vi "Line+Scan_Y.vi"() -> ()   [LabVIEW 2014]
doc: "This is the main user interface of the Raman spectroscopy system."
uses:
  <userlib>/atmcd64d.llb/AcquisitionMode_mode typedef.ctl
  <userlib>/atmcd64d.llb/ReadMode_mode typedef.ctl
  <userlib>/atmcd64d.llb/Shutter_mode typedef.ctl
  <userlib>/atmcd64d.llb/Shutter_type typedef.ctl
  <userlib>/atmcd64d.llb/TriggerMode_mode typedef.ctl
  TypeDef/GalvoInput.ctl
  <userlib>/atmcd64d.llb/Error Code Enum typedef.ctl
  TypeDef/States.ctl
panel:
  in  "Tab Control":enum32{"Main", "Andor", "Galvo"}(tab)
  in  "Galvo Center":bool
  out "Galvo":bool
  in  "Quit":bool
  out "Initialization finished":bool
  in  "Galvo Stop":bool
  in  "Galvo Scan":bool
  out "Andor":bool
  out "CurrentFrame":i32
  in  "Scan parameters":T1={"area/um"=10.2262, "range_x/v"=0.17651, "range_y/v"=0.2155, "interval/um"=0.15978, "x_center/v"=3.35, "y_center/v"=5.55, "theta_1/de"=0.0, "theta_2/de"=60.0, "theta_3/de"=120.0}
  in  "Set":bool
  in  "AndorSnap":bool
  out "SaveStatus":bool
  in  "FilePath":string="C:\\Users\\light\\Desktop\\SI+Raman\\data\\TEMP"
  in  "Exit":bool
  out "ShutDown":cluster{"CoolOff":bool, "ShutDown":bool}
  in  "Mode":T7={"AcqMode"=enum."Single Scan", "ReadMode"=enum."Image", "ShutterMode"=enum."Auto", "GateMode"=enum."TTL High", "TriggerMode"=enum."Internal"}
  in  "AcqSet":T8={"openingtime"=0, "closingtime/ms"=10, "ExposureTime/s"=10.0, "AccumCycTime"=0.0, "AccumCycNum"=1, "KineticNum"=1, "KineticTime"=0.0} {"KineticTime" format="%.5f"; "AccumCycNum" format="%.5f"; "AccumCycTime" format="%.5f"; "ExposureTime/s" format="%.5f"; "closingtime/ms" format="%.2f"; "openingtime" format="%.2f"}
  out "Timing":T9 {"kinetic" format="%.7f"; "accumulate" format="%.7f"; "exposure" format="%.7f"}
  out "SetOut":T10
  in  "MultiTrack":cluster{"StartRow":i32, "EndRow":i32}={"StartRow"=131, "EndRow"=143}
  out "SetStatus":bool
  out "CurrentTemp":i32
  out "DevInit":bool
  out "DevSize":cluster{"xpixels":i32, "ypixels":i32}
  out "HardWVersion":T11
  out "SoftWVersion":T12
  out "Speeds":T13
  in  "TargetTemp":i32=-60
  out "CoolerON":T14
  out "GetStatus":T15
  in  "YOffset":dbl=5.75 caption="Offset"
  in  "XOffset":dbl=3.1 caption="Offset"
  out "Sample Rate":dbl=1000.0 format="%0.2f"
  out "Waveform Graph":waveform(dbl)[](graph)=[{"t0"=timestamp(0 s since 1904-01-01), "dt"=0.001, "Y"=[]}]
  in  "ZOffset":dbl=1.6 caption="Offset"
  in  "Galvo":T16={"Sample Rate"=1000000.0, "Sample Clock Source"="OnboardClock", "Max Voltage"=10.0, "Min Voltage"=-10.0, "Physical Channel(s)"="Dev1/ao0,Dev1/ao1,Dev1/ao3"}
  in  "Reset":bool
  # "Objective: CFI Plan Fluor ELWD 60x (1.27 NA) \nThe depth of field: 1.78 um\nPixel Size: 0.0877um/px"
  # "Kinetics->SignleTrack"
  # "Galvo Control"
  # "10^4->1s"
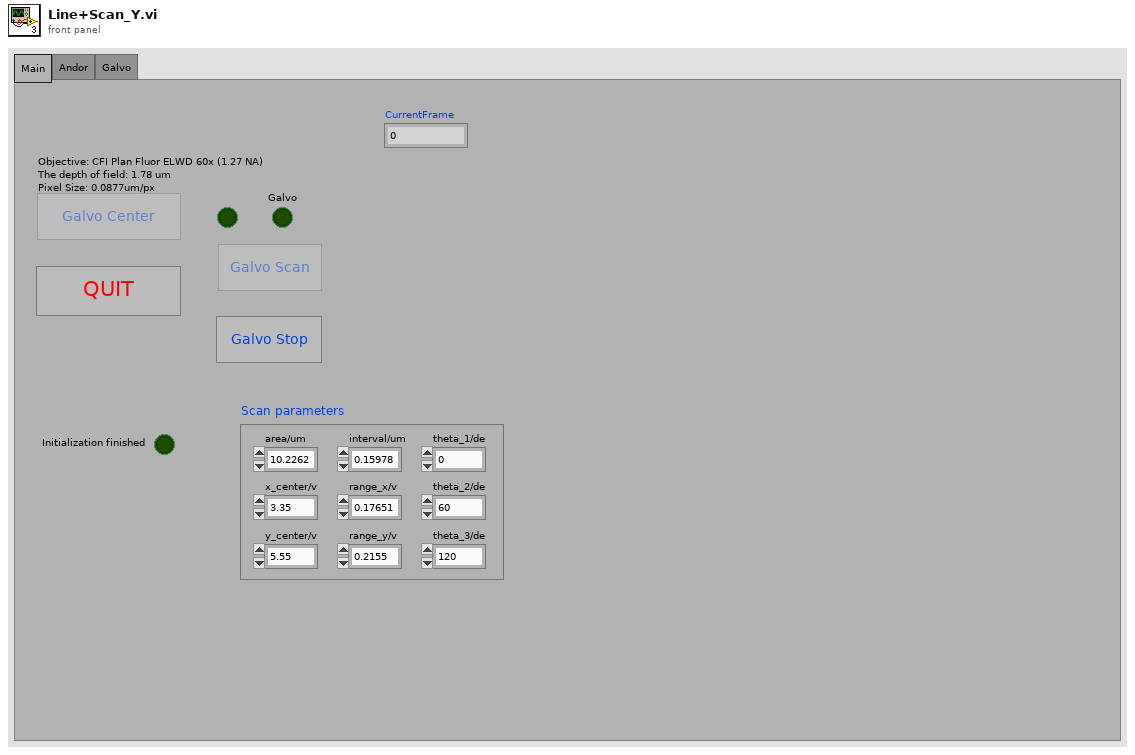
[diagram p1: front panel]
types:
  T1 = cluster{"area/um":dbl, "range_x/v":dbl, "range_y/v":dbl, "interval/um":dbl, "x_center/v":dbl, "y_center/v":dbl, "theta_1/de":dbl, "theta_2/de":dbl, "theta_3/de":dbl}
  T2 = typedef "AcquisitionMode_mode typedef.ctl" = enum16{"Reserved (0)", "Single Scan", "Accumulate", "Kinetics", "Fast Kinetics", "Run Till Abort", "Reserved (6)", "Reserved (7)", "Reserved (8)", "Time Delayed Integration"}
  T3 = typedef "ReadMode_mode typedef.ctl" = enum16{"Full Vertical Binning", "Multi-Track", "Random-Track", "Single-Track", "Image"}
  T4 = typedef "Shutter_mode typedef.ctl" = enum16{"Auto", "Open", "Close", "N/A (3)", "Open FVB Series", "Open Any Series"}
  T5 = typedef "Shutter_type typedef.ctl" = enum16{"TTL Low", "TTL High"}
  T6 = typedef "TriggerMode_mode typedef.ctl" = enum16{"Internal", "External", "N/A (2)", "N/A (3)", "N/A (4)", "N/A (5)", "External Start", "External Exposure (Bulb)", "N/A (8)", "External FVB EM", "Software", "N/A (11)", "External Charge Shifting"}
  T7 = cluster{"AcqMode":T2, "ReadMode":T3, "ShutterMode":T4, "GateMode":T5, "TriggerMode":T6}
  T8 = cluster{"openingtime":i32, "closingtime/ms":i32, "ExposureTime/s":sgl, "AccumCycTime":sgl, "AccumCycNum":i32, "KineticNum":i32, "KineticTime":sgl}
  T9 = cluster{"exposure":sgl, "accumulate":sgl, "kinetic":sgl}
  T10 = cluster{"Height":i32, "Width":i32, "bottom":i32, "gap":i32}
  T11 = cluster{"PCB":u32, "Flex":u32, "dummy1":u32, "dummy2":u32, "dummy3":u32, "dummy4":u32}
  T12 = cluster{"eprom":u32, "cofFile":u32, "vxdRev":u32, "vxdVer":u32, "dllRev":u32, "dllVer":u32}
  T13 = cluster{"NVS":i32, "VS":i32, "NHS":dbl, "HS":i32}
  T14 = cluster{"SetTemp":bool, "CoolerOn":bool, "Stablized":bool}
  T15 = cluster{"GetDetector":bool, "GetHardVer":bool, "GetNVS":bool, "GetVS":bool, "GetSotfVer":bool, "GetNHS":bool, "GetHS":bool}
  T16 = typedef "GalvoInput.ctl" = cluster{"Sample Rate":dbl, "Sample Clock Source":tag, "Max Voltage":dbl, "Min Voltage":dbl, "Physical Channel(s)":tag}
  T17 = typedef "States.ctl" = enum16{"Initialize", "CMOS live", "Shut down"}
  T18 = enum8{"Enabled", "Disabled", "Disabled and Grayed Out"}
  T19 = typedef "Error Code Enum typedef.ctl" = enum32{"N/A (0)", "DRV_ERROR_CODES", "DRV_SUCCESS", "DRV_VXDNOTINSTALLED", "DRV_ERROR_SCAN", "DRV_ERROR_CHECK_SUM", "DRV_ERROR_FILELOAD", "DRV_UNKNOWN_FUNC", "DRV_ERROR_VXD_INIT", "DRV_ERROR_ADDRESS", "DRV_ERROR_PAGELOCK", "DRV_ERROR_PAGEUNLOCK", "DRV_ERROR_BOARDTEST", "DRV_ERROR_ACK", "DRV_ERROR_UP_FIFO", "DRV_ERROR_PATTERN", "N/A (16)", "DRV_ACQUISITION_ERRORS", "DRV_ACQ_BUFFER", "DRV_ACQ_DOWNFIFO_FULL", "DRV_PROC_UNKONWN_INSTRUCTION", "DRV_ILLEGAL_OP_CODE", "DRV_KINETIC_TIME_NOT_MET", "DRV_ACCUM_TIME_NOT_MET", "DRV_NO_NEW_DATA", "N/A (25)", "DRV_SPOOLERROR", "N/A (27)", "N/A (28)", "N/A (29)", "N/A (30)", "N/A (31)", "N/A (32)", "DRV_TEMPERATURE_CODES", "DRV_TEMPERATURE_OFF", "DRV_TEMPERATURE_NOT_STABILIZED", "DRV_TEMPERATURE_STABILIZED", "DRV_TEMPERATURE_NOT_REACHED", "DRV_TEMPERATURE_OUT_RANGE", "DRV_TEMPERATURE_NOT_SUPPORTED", "DRV_TEMPERATURE_DRIFT", "N/A (41)", "N/A (42)", "N/A (43)", "N/A (44)", "N/A (45)", "N/A (46)", "N/A (47)", "N/A (48)", "DRV_GENERAL_ERRORS", "DRV_INVALID_AUX", "DRV_COF_NOTLOADED", "DRV_FPGAPROG", "DRV_FLEXERROR", "DRV_GPIBERROR", "N/A (55)", "N/A (56)", "N/A (57)", "N/A (58)", "N/A (59)", "N/A (60)", "N/A (61)", "N/A (62)", "N/A (63)", "DRV_DATATYPE", "DRV_DRIVER_ERRORS", "DRV_P1INVALID", "DRV_P2INVALID", "DRV_P3INVALID", "DRV_P4INVALID", "DRV_INIERROR", "DRV_COFERROR", "DRV_ACQUIRING", "DRV_IDLE", "DRV_TEMPCYCLE", "DRV_NOT_INITIALIZED", "DRV_P5INVALID", "DRV_P6INVALID", "DRV_INVALID_MODE", "DRV_INVALID_FILTER", "DRV_I2CERRORS", "DRV_I2CDEVNOTFOUND", "DRV_I2CTIMEOUT", "DRV_P7INVALID", "N/A (84)", "N/A (85)", "N/A (86)", "N/A (87)", "N/A (88)", "N/A (89)", "DRV_IOCERROR", "DRV_VRMVERSIONERROR"}
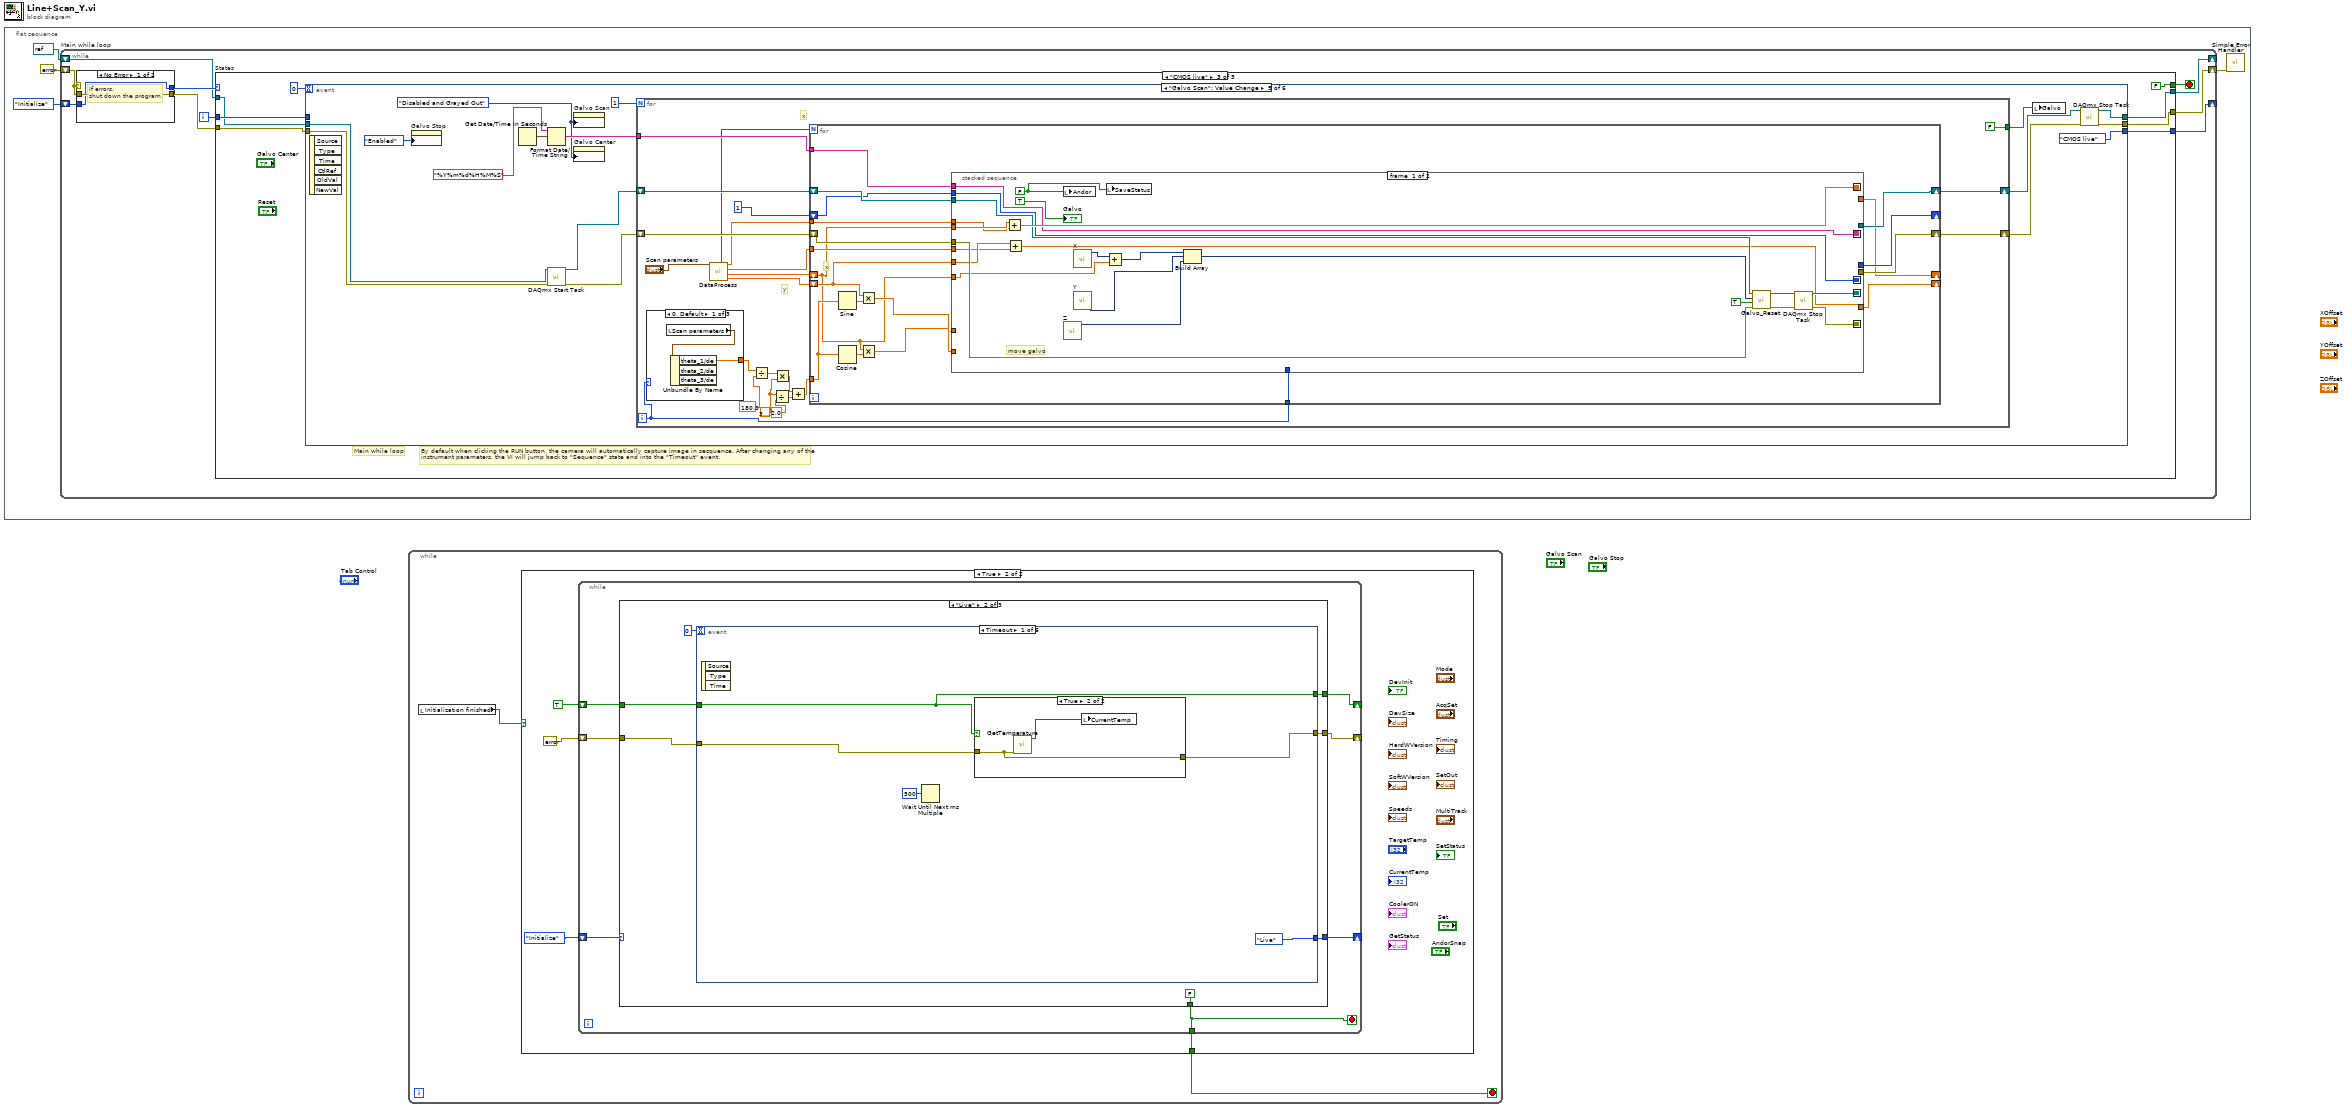
[diagram p0: block diagram]
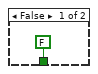
[diagram p2: hidden frame]
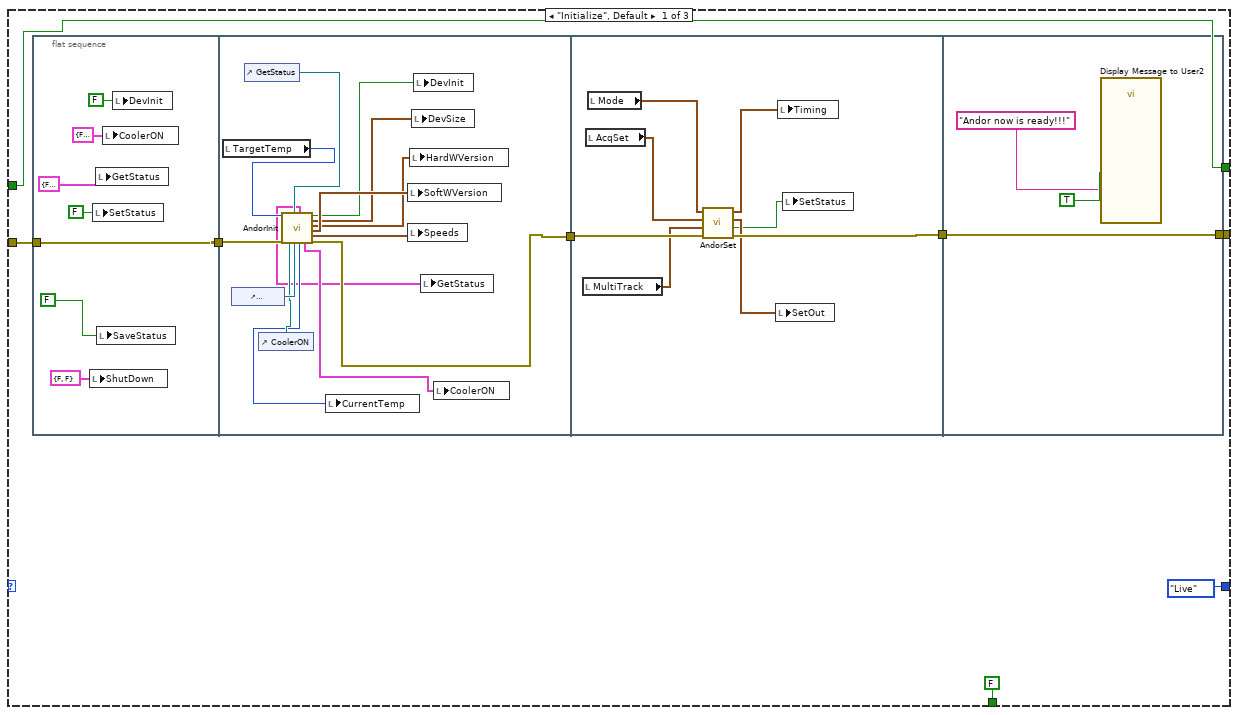
[diagram p3: hidden frame]
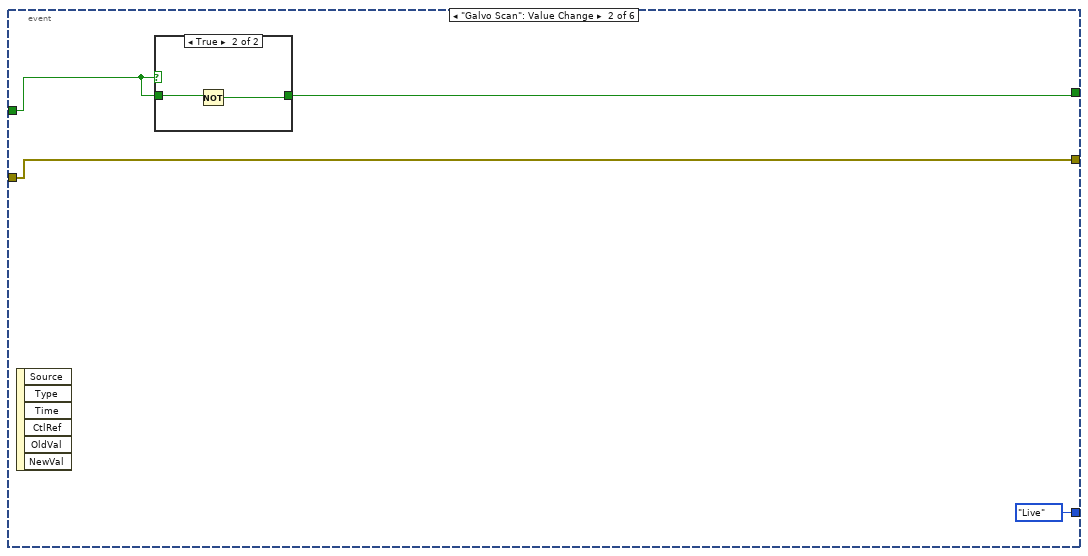
[diagram p5: hidden frame]
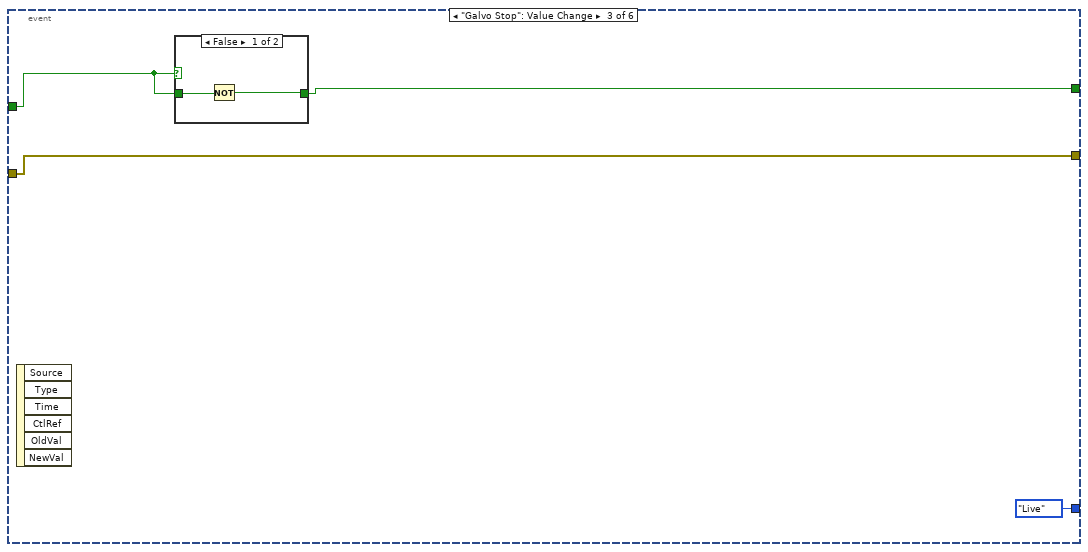
[diagram p7: hidden frame]
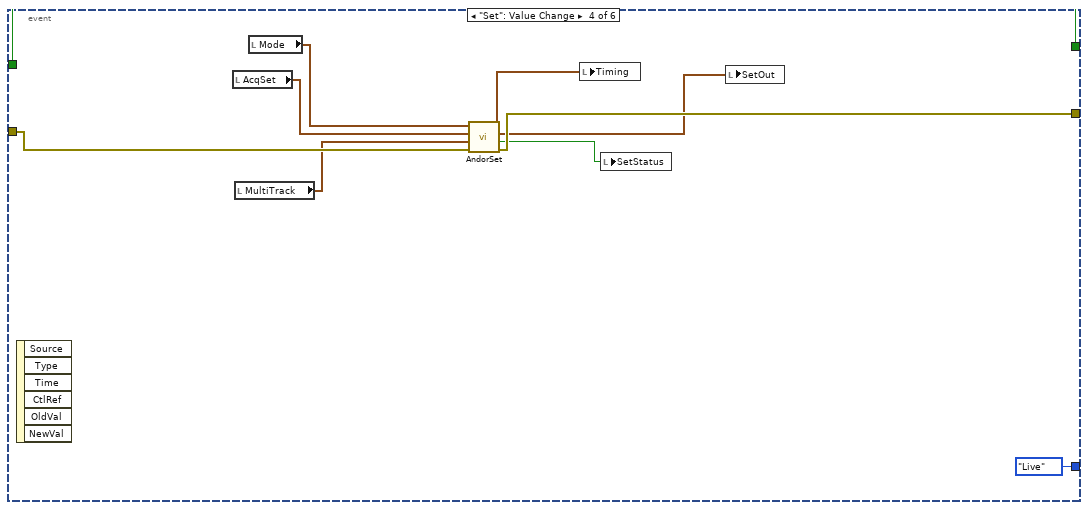
[diagram p9: hidden frame]
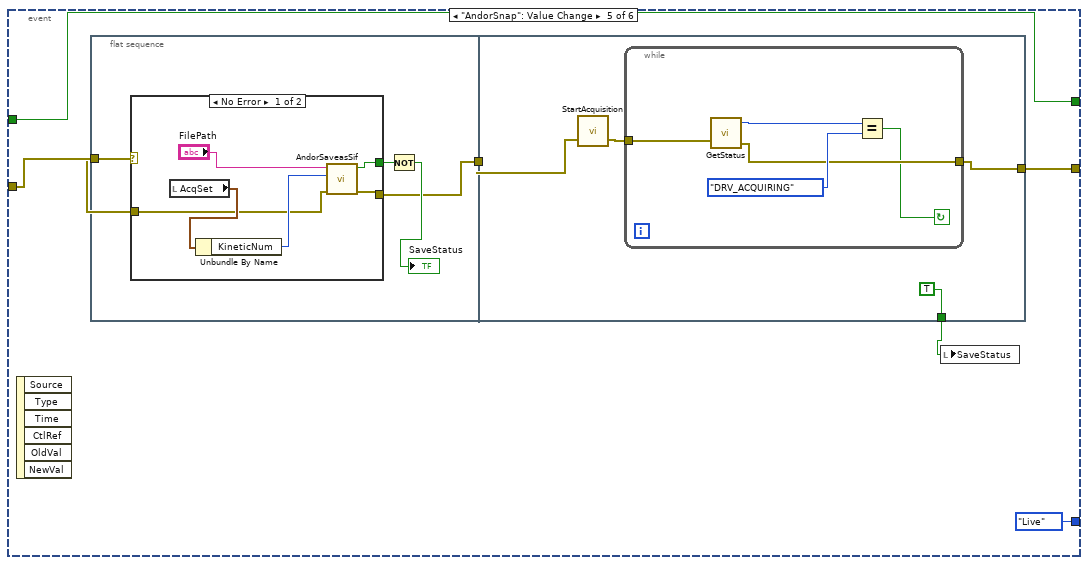
[diagram p10: hidden frame]
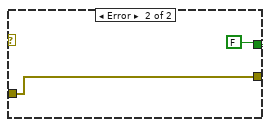
[diagram p11: hidden frame]
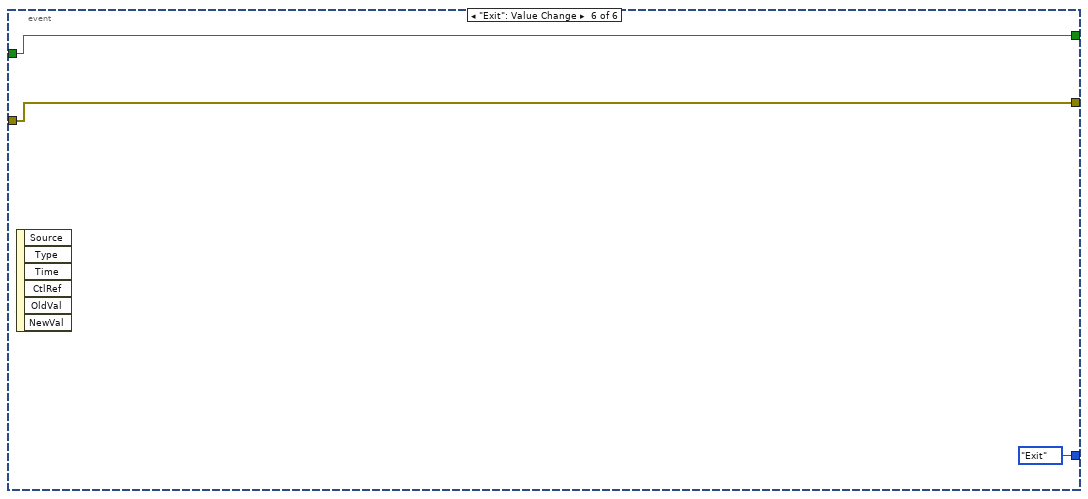
[diagram p12: hidden frame]
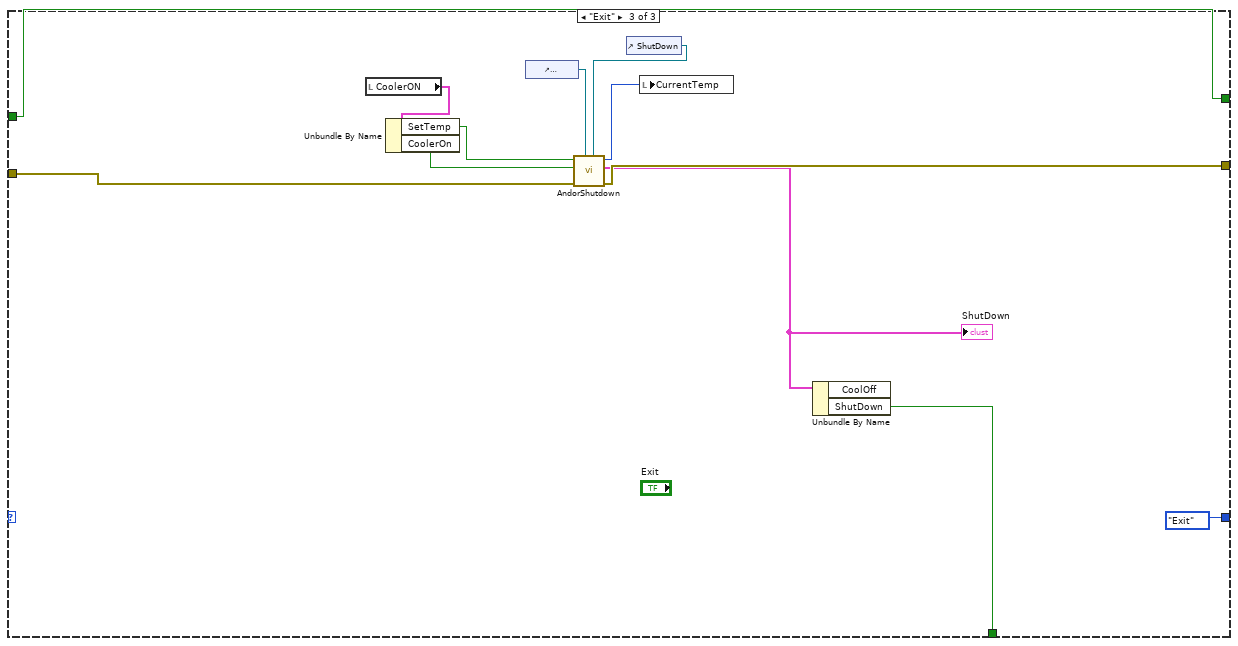
[diagram p13: hidden frame]
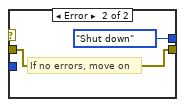
[diagram p14: hidden frame]
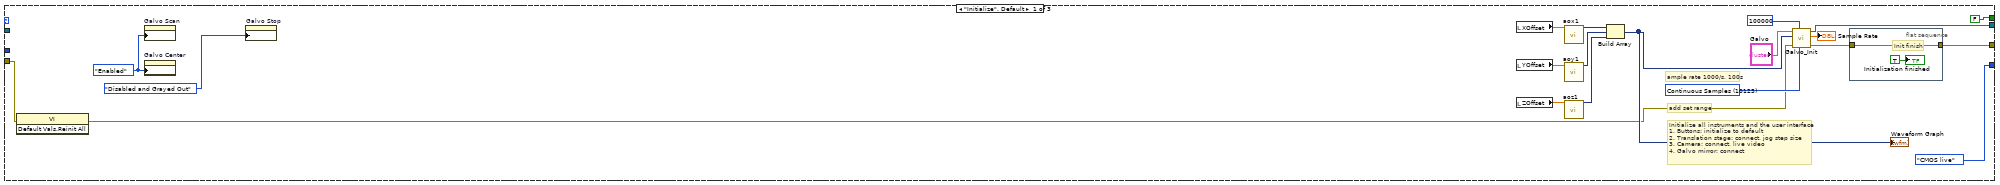
[diagram p15: hidden frame]
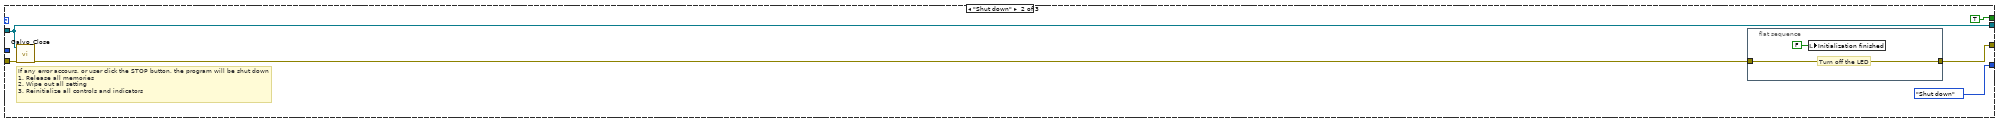
[diagram p16: hidden frame]
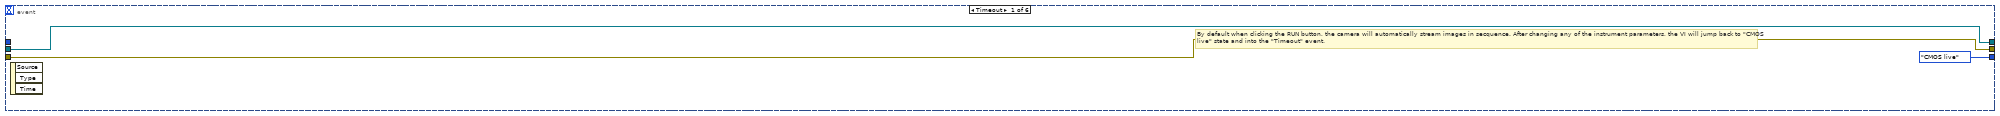
[diagram p17: hidden frame]
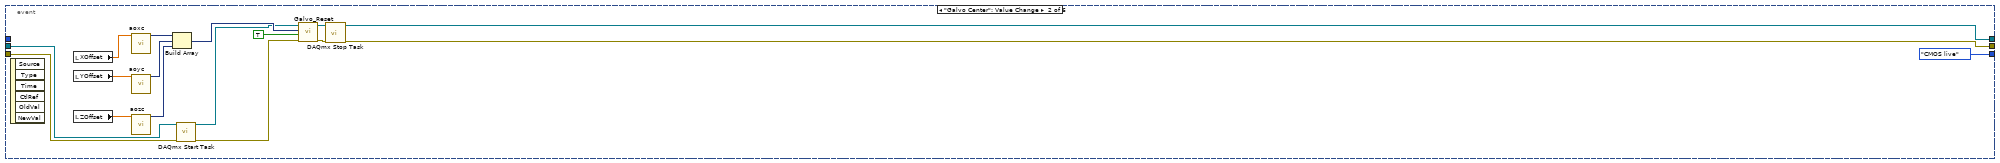
[diagram p18: hidden frame]
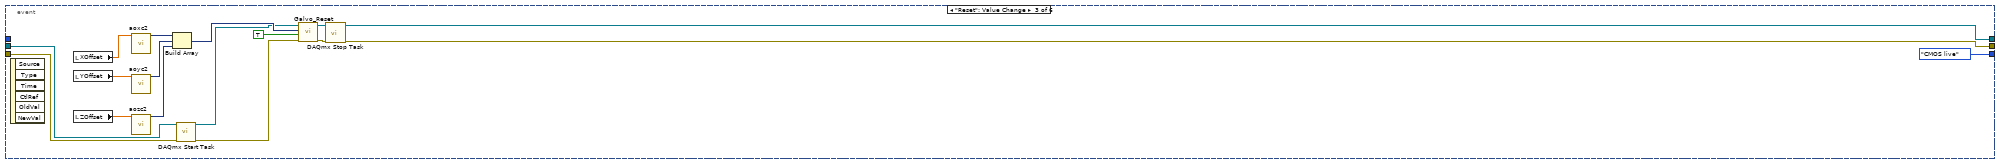
[diagram p19: hidden frame]
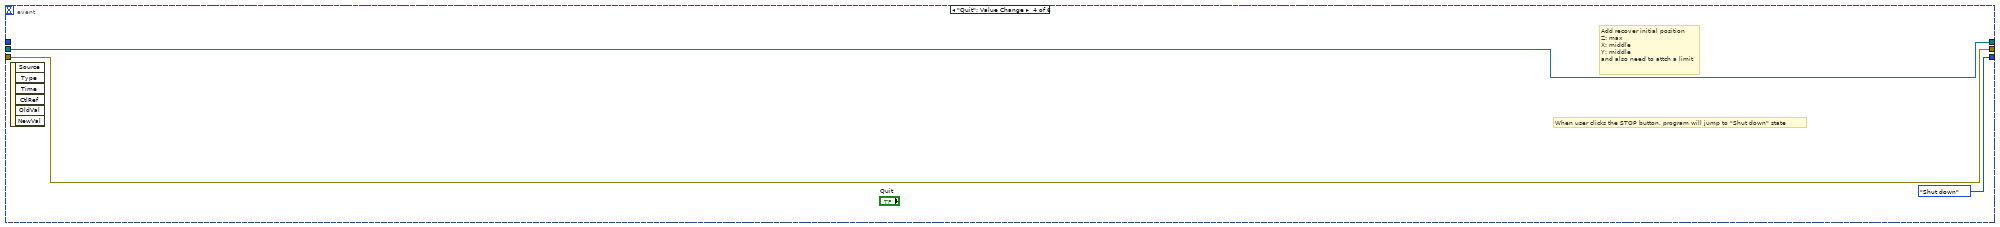
[diagram p20: hidden frame]
diagram:
  n1 = flat-sequence {
    frame #0 {
      n2 = while "Main while loop" {
        shift-right: [w9] -> _
        shift-left: States."Initialize" -> [w14]
        shift-right: [w12] -> w2
        shift-left: errorcluster {"status"=FALSE, "code"=0, "source"=""} ("error out") -> [w8]
        shift-right: [w6] -> _
        shift-left: refnum<k21> refnum ("task out") -> [w5]
        i -> [w7]
        stop <- w10 stop-if-true
        n3 = case shown="No Error" w8 {
          tunnel: w8 -> [w16 w18]
          tunnel: [w16 w18] -> w11
          tunnel: w14 -> [w15 _]
          tunnel: [w15 States."Shut down"] -> w13
          frame No Error {
            # "If errors,\nshut down the program"
          }
          frame Error {
            # "If no errors, move on"
          }
        }
        n4 = case "States" shown="\"CMOS live\"" w13 {
          tunnel: [w36 w41 w54] -> w12
          tunnel: w11 -> [w37 w42 w55]
          tunnel: [FALSE TRUE FALSE] -> w10
          tunnel: [States."CMOS live" States."Shut down" w56] -> w9
          tunnel: w7 -> [_ _ w52]
          tunnel: [w33 w44 w50] -> w6
          tunnel: w5 -> [_ w44 w51]
          frame "Initialize", Default {
            w22 = T18."Enabled" ("Disabled")
            w28 = 10123 items=["Finite Samples"=10178, "Continuous Samples"=10123, "Hardware Timed Single Point"=12522] ("Sample Mode")
            # "ample rate 1000/s, 100s"
            # "add set range"
            # "Initialize all instruments and the user interface\n1. Buttons: initialize to default\n2. Translation stage: connect, jog step size\n3. Camera: connect, live video\n4. Galvo mirror: connect"
            n5 = invoke class="VI" method="Default Vals.Reinit All"(error in=w37) -> (error out=w21:errorcluster)  [unwired: 2 in, 2 out]
            n6 = property on="Galvo Scan" class="Bool"("DisabledEnum"=w22) -> ()  [unwired: 2 in, 2 out]
            n7 = property on="Galvo Center" class="Bool"("DisabledEnum"=w22) -> ()  [unwired: 2 in, 2 out]
            n8 = property on="Galvo Stop" class="Bool"("DisabledEnum"=T18."Disabled and Grayed Out" ("Disabled")) -> ()  [unwired: 2 in, 2 out]
            n9 = local read "XOffset"() -> (w25:dbl)
            n10 = local read "YOffset"() -> (w24:dbl)
            n11 = local read "ZOffset"() -> (w23:dbl)
            n12 = call "aox1"("Offset"=w25) -> ("DC"=w27:dynamicdata)  [unwired: 13 in, 1 out]
            n13 = call "aoy1"("Offset"=w24) -> ("DC"=w26:dynamicdata)  [unwired: 13 in, 1 out]
            n14 = call "aoz1"("Offset"=w23) -> ("DC"=w31:dynamicdata)  [unwired: 13 in, 1 out]
            n15 = Build Array(w27, w26, w31) -> (w30:dynamicdata[])
            "Waveform Graph" <- w30
            n16 = call "Galvo_Init.vi"("Sample Mode"=w28, "samples per channel"=100000, "error in"=w21, "Signal array"=w30, "Galvo_Input"="Galvo") -> ("error out"=w32:errorcluster, "Actual Sample Rate"=→"Sample Rate":dbl, "task out"=w33:refnum<k21>)  [unwired: 4 in]
            n17 = flat-sequence {
              tunnel: w32 -> [w40]
              tunnel: [w40] -> w36
              frame #0 {
                # "Init finish"
                "Initialization finished" <- TRUE ("Initialization finished")
              }
            }
          }
          frame "Shut down" {
            # "If any error accours, or user click the STOP button, the program will be shut down\n1. Release all memories\n2. Wipe out all setting\n3. Reinitialize all controls and indicators"
            n18 = call "Galvo_Close.vi"("error in"=w42, "task/channels in"=w44) -> ("error out"=w43:errorcluster)  [unwired: 9 in]
            n19 = flat-sequence {
              tunnel: w43 -> [w47]
              tunnel: [w47] -> w41
              frame #0 {
                # "Turn off the LED"
                n20 = local write "Initialization finished"(FALSE ("Initialization finished")) -> ()
              }
            }
          }
          frame "CMOS live" {
            # "Main while loop"
            # "By default when clicking the RUN button, the camera will automatically capture image in secquence. After changing any of the \ninstrument parameters, the VI will jump back to \"Sequence\" state and into the \"Timeout\" event."
            n21 = event shown="[4] \"Galvo Scan\": Value Change" {
              selector: _ -> [_ _ _ _ _ _]
              dyn-events: _ -> [_ _ _ _ _ _]
              timeout: 0 -> [_ _ _ _ _ _]
              tunnel: [States."CMOS live" States."CMOS live" States."CMOS live" States."Shut down" States."CMOS live" States."CMOS live"] -> w56
              tunnel: w55 -> [w57 w68 w85 w95 w100 w237]
              tunnel: [w57 w62 w79 w95 w105 w237] -> w54
              tunnel: w52 -> [_ _ _ _ _ _]
              tunnel: [w59 w63 w80 w94 w104 w239] -> w50
              tunnel: w51 -> [w59 w70 w87 w94 w111 w239]
              event Timeout {
                # "By default when clicking the RUN button, the camera will automatically stream images in secquence. After changing any of the instrument parameters, the VI will jump back to \"CMOS live\" state and into the \"Timeout\" event."
                n22 = event-data() -> ()  [unwired: 1 in, 3 out]
              }
              event "Galvo Center": Value Change {
                n23 = event-data() -> ()  [unwired: 1 in, 6 out]
                n24 = local read "XOffset"() -> (w61:dbl)
                n25 = local read "YOffset"() -> (w60:dbl)
                n26 = local read "ZOffset"() -> (w74:dbl)
                n27 = call "aoxc"("Offset"=w61) -> ("DC"=w72:dynamicdata)  [unwired: 13 in, 1 out]
                n28 = call "aoyc"("Offset"=w60) -> ("DC"=w71:dynamicdata)  [unwired: 13 in, 1 out]
                n29 = call "aozc"("Offset"=w74) -> ("DC"=w75:dynamicdata)  [unwired: 13 in, 1 out]
                n30 = Build Array(w72, w71, w75) -> (w73:dynamicdata[])
                n31 = call <vilib>:"DAQmx Start Task.vi"("task/channels in"=w70, "error in"=w68) -> ("task out"=w69:refnum<k21>, "error out"=w67:errorcluster)  [unwired: 12 in]
                n32 = call "Galvo_Reset.vi"("error in"=w67, "auto start"=TRUE, "Signal array"=w73, "task/channels in"=w69) -> ("error out"=w64:errorcluster, "task out"=w65:refnum<k21>)  [unwired: 6 in]
                n33 = call <vilib>:"DAQmx Stop Task.vi"("task/channels in"=w65, "error in"=w64) -> ("task out"=w63:refnum<k21>, "error out"=w62:errorcluster)  [unwired: 12 in]
              }
              event "Reset": Value Change {
                n34 = event-data() -> ()  [unwired: 1 in, 6 out]
                n35 = local read "XOffset"() -> (w78:dbl)
                n36 = local read "YOffset"() -> (w77:dbl)
                n37 = local read "ZOffset"() -> (w91:dbl)
                n38 = call "aoxc2"("Offset"=w78) -> ("DC"=w89:dynamicdata)  [unwired: 13 in, 1 out]
                n39 = call "aoyc2"("Offset"=w77) -> ("DC"=w88:dynamicdata)  [unwired: 13 in, 1 out]
                n40 = call "aozc2"("Offset"=w91) -> ("DC"=w92:dynamicdata)  [unwired: 13 in, 1 out]
                n41 = Build Array(w89, w88, w92) -> (w90:dynamicdata[])
                n42 = call <vilib>:"DAQmx Start Task.vi"("task/channels in"=w87, "error in"=w85) -> ("task out"=w86:refnum<k21>, "error out"=w84:errorcluster)  [unwired: 12 in]
                n43 = call "Galvo_Reset.vi"("error in"=w84, "auto start"=TRUE, "Signal array"=w90, "task/channels in"=w86) -> ("error out"=w81:errorcluster, "task out"=w82:refnum<k21>)  [unwired: 6 in]
                n44 = call <vilib>:"DAQmx Stop Task.vi"("task/channels in"=w82, "error in"=w81) -> ("task out"=w80:refnum<k21>, "error out"=w79:errorcluster)  [unwired: 12 in]
              }
              event "Quit": Value Change {
                # "Add recover initial position\nZ: max\nX: middle\nY: middle\nand also need to attch a limit"
                # "When user clicks the STOP button, program will jump to \"Shut down\" state"
                n45 = event-data() -> ()  [unwired: 1 in, 6 out]
              }
              event "Galvo Scan": Value Change {
                w98 = T18."Disabled and Grayed Out" ("Disabled")
                n46 = event-data() -> ()  [unwired: 1 in, 6 out]
                n47 = property on="Galvo Stop" class="Bool"("DisabledEnum"=T18."Enabled" ("Disabled")) -> ()  [unwired: 2 in, 2 out]
                n48 = Get Date/Time In Seconds() -> (seconds since 1Jan1904=w103:timestamp)
                n49 = Format Date/Time String(time format string (%c)="%Y%m%d%H%M%S", seconds (now)=w103) -> (date/time string=w101:string)  [unwired: 1 in]
                n50 = call <vilib>:"DAQmx Start Task.vi"("task/channels in"=w111, "error in"=w100) -> ("task out"=w108:refnum<k21>, "error out"=w110:errorcluster)  [unwired: 12 in]
                n51 = property on="Galvo Scan" class="Bool"("DisabledEnum"=w98) -> ()  [unwired: 2 in, 2 out]
                n52 = property on="Galvo Center" class="Bool"("DisabledEnum"=w98) -> ()  [unwired: 2 in, 2 out]
                n53 = for {
                  N: 1 -> [_]
                  tunnel: [FALSE ("Galvo")] -> w109
                  shift-right: [w133] -> w106
                  shift-left: w110 -> [w132]
                  shift-right: [w130] -> w107
                  shift-left: w108 -> [w131]
                  tunnel: w101 -> [w129]
                  i -> [w120]
                  w124 = 3.141592653589793
                  # "y"
                  # "x"
                  n54 = case shown="0, Default" w120 {
                    tunnel: [w135 w137 w139] -> w127
                    frame 0, Default {
                      n55 = local read "Scan parameters"() -> (w136:T1)
                      n56 = Unbundle By Name(w136) -> ("theta_1/de"=w135:dbl)  [unwired: 2 out]
                    }
                    frame 1 {
                      n57 = local read "Scan parameters"() -> (w138:T1)
                      n58 = Unbundle By Name(w138) -> ("theta_2/de"=w137:dbl)  [unwired: 2 out]
                    }
                    frame 2 {
                      n59 = local read "Scan parameters"() -> (w140:T1)
                      n60 = Unbundle By Name(w140) -> ("theta_3/de"=w139:dbl)  [unwired: 2 out]
                    }
                  }
                  n61 = call "DataProcess.vi"("Scan parameters"="Scan parameters") -> ("ystart"=w115:dbl, "xstart"=w116:dbl, "ystep"=w113:dbl, "xstep"=w114:dbl, "NUM"=w117:i32)  [unwired: 6 in]
                  n62 = Divide(x=w127, y=180.0 ("x")) -> (x/y=w126:dbl)
                  n63 = Divide(x=w124, y=2.0) -> (x/y=w123:dbl)
                  n64 = Multiply(x=w126, y=w124) -> (x*y=w125:dbl)
                  n65 = Add(x=w125, y=w123) -> (x+y=w121:dbl)
                  n66 = for {
                    N: w117 -> [_]
                    shift-right: [w154] -> w133
                    shift-left: w132 -> [w159]
                    shift-right: [w155] -> w130
                    shift-left: w131 -> [w158]
                    shift-right: [w153] -> _
                    shift-left: 1 -> [w157]
                    tunnel: w129 -> [w156]
                    tunnel: w121 -> [w152]
                    shift-right: [w149] -> _
                    shift-left: w116 -> [w141]
                    shift-right: [w150] -> _
                    shift-left: w115 -> [w144]
                    tunnel: w120 -> [w151]
                    tunnel: w114 -> [w148]
                    tunnel: w113 -> [w147]
                    # "x"
                    n67 = Sine(x=w152) -> (sin(x)=w145:dbl)
                    n68 = Cosine(x=w152) -> (cos(x)=w146:dbl)
                    n69 = Multiply(x=w144, y=w145) -> (x*y=w143:dbl)
                    n70 = Multiply(x=w141, y=w146) -> (x*y=w142:dbl)
                    n71 = stacked-sequence {
                      seq-local: [w177 _] -> [_ w188]
                      seq-local: [w179 _] -> [_ w189]
                      seq-local: [w175 _] -> [_ w194]
                      seq-local: [w174 _] -> [_ w187]
                      seq-local: [w171 _] -> [_ w186]
                      tunnel: w159 -> [w180 _]
                      tunnel: w158 -> [w173 _]
                      tunnel: w157 -> [w175 _]
                      tunnel: w156 -> [w174 _]
                      tunnel: [_ w189] -> w149
                      tunnel: [_ w192] -> w153
                      tunnel: [_ w191] -> w154
                      tunnel: [_ w184] -> w155
                      tunnel: w142 -> [_ _]
                      tunnel: w143 -> [_ _]
                      tunnel: w141 -> [w170 _]
                      tunnel: w144 -> [w169 _]
                      tunnel: [w168 _] -> w150
                      tunnel: w151 -> [_ w183]
                      tunnel: w148 -> [w166 _]
                      tunnel: w147 -> [w165 _]
                      tunnel: w141 -> [w160 _]
                      frame #0 {
                        w182 = FALSE ("SaveStatus")
                        # "move galvo"
                        n72 = Add(x=w170, y=w166) -> (x+y=w179:dbl)
                        n73 = Add(x=w169, y=w165) -> (x+y=w168:dbl)
                        n74 = local write "Andor"(w182) -> ()
                        n75 = call "Z"() -> ("Signal"=w167:dynamicdata)  [unwired: 9 in, 2 out]
                        n76 = call "X"() -> ("Signal"=w162:dynamicdata)  [unwired: 9 in, 2 out]
                        n77 = call "Y"() -> ("Signal"=w163:dynamicdata)  [unwired: 9 in, 2 out]
                        n78 = local write "SaveStatus"(w182) -> ()
                        n79 = Add(x=w162, y=w160) -> (x+y=w161:dynamicdata)
                        n80 = Build Array(w161, w163, w167) -> (w164:dynamicdata[])
                        n81 = call "Galvo_Reset.vi"("error in"=w180, "auto start"=TRUE, "Signal array"=w164, "task/channels in"=w173) -> ("error out"=w178:errorcluster, "task out"=w172:refnum<k21>)  [unwired: 6 in]
                        n82 = call <vilib>:"DAQmx Stop Task.vi"("task/channels in"=w172, "error in"=w178) -> ("task out"=w171:refnum<k21>, "error out"=w177:errorcluster)  [unwired: 12 in]
                        "Galvo" <- TRUE
                      }
                      frame #1 {
                        n83 = flat-sequence {
                          tunnel: [w203] -> w195
                          tunnel: w194 -> [w201]
                          tunnel: [w200] -> w193
                          tunnel: w188 -> [w199]
                          tunnel: w187 -> [w198]
                          tunnel: w186 -> [w197]
                          tunnel: [w197] -> w185
                          tunnel: w183 -> [w196]
                          tunnel: [w223] -> w191
                          tunnel: w195 -> [w221]
                          tunnel: w193 -> [w222]
                          tunnel: [w222] -> w192
                          tunnel: [FALSE ("Galvo")] -> w190
                          tunnel: w185 -> [w219]
                          tunnel: [w218] -> w184
                          frame #0 {
                            n84 = case shown="Error" w199 {
                              tunnel: [w213 w215] -> w203
                              tunnel: [w212 w216] -> w200
                              tunnel: [w211 FALSE ("SaveStatus")] -> w202
                              tunnel: w201 -> [w210 w216]
                              tunnel: w199 -> [w207 w215]
                              tunnel: w198 -> [w206 _]
                              tunnel: w196 -> [w204 _]
                              frame No Error {
                                n85 = local read "AcqSet"() -> (w209:T8)
                                n86 = Unbundle By Name(w209) -> ("KineticNum"=w208:i32)
                                n87 = local read "FilePath"() -> (w214:string)
                                n88 = Increment(x=w210) -> (x+1=w212:i32)
                                n89 = call "AndorSaveasSif_Ver2.vi"("Phase"=0, "Time"=w206, "Dir"=w204, "error in"=w207, "No."=w210, "KinNumber"=w208, "FilePath"=w214) -> ("error out"=w213:errorcluster, "SaveStatus"=w211:bool)  [unwired: 3 in]
                                "CurrentFrame" <- w210
                              }
                              frame Error {
                              }
                            }
                            n90 = local write "SaveStatus"(w202) -> ()
                          }
                          frame #1 {
                            n91 = flat-sequence {
                              tunnel: [w231] -> w225
                              tunnel: [TRUE] -> w224
                              tunnel: w221 -> [w229]
                              tunnel: [w227] -> w218
                              tunnel: w219 -> [w226]
                              frame #0 {
                                n92 = call <vilib>:"DAQmx Start Task.vi"("task/channels in"=w226, "error in"=w229) -> ("task out"=w227:refnum<k21>, "error out"=w228:errorcluster)  [unwired: 12 in]
                                n93 = call <userlib>:"StartAcquisition.vi"("error in (no error)"=w228) -> ("error out"=w231:errorcluster)  [unwired: 1 in, 1 out]
                              }
                            }
                            n94 = local write "Andor"(w224) -> ()
                            n95 = while {
                              tunnel: w225 -> [w236]
                              tunnel: [w233] -> w223
                              stop <- w232 continue-if-true
                              n96 = call <userlib>:"GetStatus.vi"("error in (no error)"=w236) -> ("error out"=w233:errorcluster, "status"=w235:T19)  [unwired: 2 in, 1 out]
                              n97 = Equal?(x=Error_Code_Enum_typedef."DRV_ACQUIRING" ("y"), y=w235) -> (x = y?=w232:bool)
                              "Andor" <- w232
                            }
                          }
                        }
                        n98 = local write "Galvo"(w190) -> ()
                      }
                    }
                  }
                }
                n99 = local write "Galvo"(w109) -> ()
                n100 = call <vilib>:"DAQmx Stop Task.vi"("task/channels in"=w107, "error in"=w106) -> ("task out"=w104:refnum<k21>, "error out"=w105:errorcluster)  [unwired: 12 in]
              }
              event "Galvo Stop": Value Change {
                (unwired) T18."Disabled and Grayed Out" ("Disabled")
                w238 = T18."Enabled" ("Disabled")
                n101 = event-data() -> ()  [unwired: 1 in, 6 out]
                n102 = property on="Galvo Scan" class="Bool"("DisabledEnum"=w238) -> ()  [unwired: 2 in, 2 out]
                n103 = property on="Galvo Center" class="Bool"("DisabledEnum"=w238) -> ()  [unwired: 2 in, 2 out]
              }
            }
          }
        }
      }
      n104 = call <vilib>:"Simple Error Handler.vi"("error in (no error)"=w2) -> ()  [unwired: 4 in, 5 out]
    }
  }
  n105 = while {
    stop <- w241 stop-if-true
    n106 = local read "Initialization finished"() -> (w242:bool)
    n107 = case shown="True" w242 {
      tunnel: [FALSE ("ShutDown") w245] -> w241
      frame False {
      }
      frame True {
        n108 = while {
          shift-right: [w253] -> _
          shift-left: enum16{"Initialize", "Live", "Exit"}."Initialize" -> [w254]
          shift-right: [w251] -> _
          shift-left: errorcluster {"status"=FALSE, "code"=0, "source"=""} ("error in") -> [w252]
          tunnel: [w250] -> w245
          shift-right: [w248] -> _
          shift-left: TRUE -> [w249]
          stop <- w250 stop-if-true
          n109 = case shown="\"Live\"" w254 {
            tunnel: [enum16{"Initialize", "Live", "Exit"}."Live" w301 enum16{"Initialize", "Live", "Exit"}."Exit"] -> w253
            tunnel: w252 -> [w260 w300 w374]
            tunnel: [w257 w299 w373] -> w251
            tunnel: [FALSE ("ShutDown") FALSE ("ShutDown") w365] -> w250
            tunnel: w249 -> [w255 w296 w364]
            tunnel: [w255 w295 w364] -> w248
            frame "Initialize", Default {
              n110 = flat-sequence {
                tunnel: [w269] -> w261
                tunnel: w260 -> [w269]
                tunnel: w261 -> [w283]
                tunnel: [w282] -> w259
                tunnel: w259 -> [w291]
                tunnel: [w290] -> w258
                tunnel: w258 -> [w294]
                tunnel: [w294] -> w257
                frame #0 {
                  n111 = local write "ShutDown"(cluster{"CoolOff":bool, "ShutDown":bool} {"CoolOff"=FALSE, "ShutDown"=FALSE} ("ShutDown")) -> ()
                  n112 = local write "SetStatus"(FALSE ("SetStatus")) -> ()
                  n113 = local write "GetStatus"(T15 {"GetDetector"=FALSE, "GetHardVer"=FALSE, "GetNVS"=FALSE, "GetVS"=FALSE, "GetSotfVer"=FALSE, "GetNHS"=FALSE, "GetHS"=FALSE} ("GetStatus")) -> ()
                  n114 = local write "SaveStatus"(FALSE ("Save")) -> ()
                  n115 = local write "CoolerON"(T14 {"SetTemp"=FALSE, "CoolerOn"=FALSE, "Stablized"=FALSE} ("CoolerON")) -> ()
                  n116 = local write "DevInit"(FALSE ("DevInit")) -> ()
                }
                frame #1 {
                  n117 = local read "TargetTemp"() -> (w278:i32)
                  n118 = control-ref of="CurrentTemp"() -> (w280:refnum<vi>)
                  n119 = control-ref of="GetStatus"() -> (w281:refnum<vi>)
                  n120 = control-ref of="CoolerON"() -> (w279:refnum<vi>)
                  n121 = call "AndorInit.vi"("TargetTemp"=w278, "error in"=w283, "CoolerONRef"=w279, "GetStatusRef"=w281, "CurrentTempRef"=w280) -> ("GetStatus"=w270:T15, "CurrentTemp"=w277:i32, "CoolerON"=w276:T14, "DevInit"=w273:bool, "DevSize"=w272:cluster{"xpixels":i32, "ypixels":i32}, "HardWVersion"=w271:T11, "SoftWVersion"=w274:T12, "Speeds"=w275:T13, "error out"=w282:errorcluster)  [unwired: 6 in]
                  n122 = local write "CurrentTemp"(w277) -> ()
                  n123 = local write "SoftWVersion"(w274) -> ()
                  n124 = local write "Speeds"(w275) -> ()
                  n125 = local write "HardWVersion"(w271) -> ()
                  n126 = local write "DevSize"(w272) -> ()
                  n127 = local write "DevInit"(w273) -> ()
                  n128 = local write "GetStatus"(w270) -> ()
                  n129 = local write "CoolerON"(w276) -> ()
                }
                frame #2 {
                  n130 = local read "MultiTrack"() -> (w287:cluster{"StartRow":i32, "EndRow":i32})
                  n131 = local read "AcqSet"() -> (w289:T8)
                  n132 = local read "Mode"() -> (w288:T7)
                  n133 = call "AndorSet.vi"("error in"=w291, "MultiTrack"=w287, "AcqSet"=w289, "Mode"=w288) -> ("error out"=w290:errorcluster, "SetStatus"=w284:bool, "SetOut"=w285:T10, "Timing"=w286:T9)  [unwired: 4 in]
                  n134 = local write "SetOut"(w285) -> ()
                  n135 = local write "Timing"(w286) -> ()
                  n136 = local write "SetStatus"(w284) -> ()
                }
                frame #3 {
                  n137 = call "Display Message to User2"("Enable"=TRUE, "Message"="Andor now is ready!!!") -> ()  [unwired: 8 in, 2 out]
                }
              }
            }
            frame "Live" {
              n138 = event shown="[0] Timeout" {
                selector: _ -> [_ _ _ _ _ _]
                dyn-events: _ -> [_ _ _ _ _ _]
                timeout: 0 -> [_ _ _ _ _ _]
                tunnel: [enum16{"Initialize", "Live", "Exit"}."Live" enum16{"Initialize", "Live", "Exit"}."Live" enum16{"Initialize", "Live", "Exit"}."Live" enum16{"Initialize", "Live", "Exit"}."Live" enum16{"Initialize", "Live", "Exit"}."Live" enum16{"Initialize", "Live", "Exit"}."Exit"] -> w301
                tunnel: w300 -> [w304 w313 w320 w332 w337 w362]
                tunnel: [w303 w313 w320 w331 w335 w362] -> w299
                tunnel: w296 -> [w302 w311 w318 w324 w334 w361]
                tunnel: [w302 w310 w317 w324 w334 w361] -> w295
                event Timeout {
                  n139 = event-data() -> ()  [unwired: 1 in, 3 out]
                  n140 = Wait Until Next ms Multiple(millisecond multiple=u32 500) -> ()  [unwired: 1 out]
                  n141 = case shown="True" w302 {
                    tunnel: w304 -> [w307 w308]
                    tunnel: [w307 w308] -> w303
                    frame False {
                    }
                    frame True {
                      n142 = call <userlib>:"GetTemperature.vi"("error in (no error)"=w308) -> ("temperature"=w309:i32)  [unwired: 3 in, 3 out]
                      n143 = local write "CurrentTemp"(w309) -> ()
                    }
                  }
                }
                event "Galvo Scan": Value Change {
                  n144 = event-data() -> ()  [unwired: 1 in, 6 out]
                  n145 = case shown="True" w311 {
                    tunnel: w311 -> [w314 w316]
                    tunnel: [w314 w315] -> w310
                    frame False {
                    }
                    frame True {
                      n146 = Not(x=w316) -> (.not. x?=w315:bool)
                    }
                  }
                }
                event "Galvo Stop": Value Change {
                  n147 = event-data() -> ()  [unwired: 1 in, 6 out]
                  n148 = case shown="False" w318 {
                    tunnel: w318 -> [w322 w323]
                    tunnel: [w321 w323] -> w317
                    frame False {
                      n149 = Not(x=w322) -> (.not. x?=w321:bool)
                    }
                    frame True {
                    }
                  }
                }
                event "Set": Value Change {
                  n150 = event-data() -> ()  [unwired: 1 in, 6 out]
                  n151 = local read "AcqSet"() -> (w329:T8)
                  n152 = local read "MultiTrack"() -> (w328:cluster{"StartRow":i32, "EndRow":i32})
                  n153 = local read "Mode"() -> (w330:T7)
                  n154 = call "AndorSet.vi"("error in"=w332, "MultiTrack"=w328, "AcqSet"=w329, "Mode"=w330) -> ("error out"=w331:errorcluster, "SetStatus"=w326:bool, "SetOut"=w325:T10, "Timing"=w327:T9)  [unwired: 4 in]
                  n155 = local write "Timing"(w327) -> ()
                  n156 = local write "SetStatus"(w326) -> ()
                  n157 = local write "SetOut"(w325) -> ()
                }
                event "AndorSnap": Value Change {
                  n158 = event-data() -> ()  [unwired: 1 in, 6 out]
                  n159 = flat-sequence {
                    tunnel: [w340] -> w338
                    tunnel: w337 -> [w343]
                    tunnel: w338 -> [w355]
                    tunnel: [TRUE ("SaveStatus")] -> w336
                    tunnel: [w352] -> w335
                    frame #0 {
                      n160 = case shown="No Error" w343 {
                        tunnel: w343 -> [w346 w351]
                        tunnel: [w345 FALSE ("SaveStatus")] -> w342
                        tunnel: [w344 w351] -> w340
                        frame No Error {
                          n161 = local read "AcqSet"() -> (w348:T8)
                          n162 = Unbundle By Name(w348) -> ("KineticNum"=w347:i32)
                          n163 = call "AndorSaveasSif.vi"("error in"=w346, "KinNumber"=w347, "FilePath"="FilePath") -> ("error out"=w344:errorcluster, "SaveStatus"=w345:bool)  [unwired: 6 in, 1 out]
                        }
                        frame Error {
                        }
                      }
                      n164 = Not(x=w342) -> (.not. x?=→"SaveStatus":bool)
                    }
                    frame #1 {
                      n165 = call <userlib>:"StartAcquisition.vi"("error in (no error)"=w355) -> ("error out"=w354:errorcluster)  [unwired: 1 in, 1 out]
                      n166 = while {
                        tunnel: w354 -> [w360]
                        tunnel: [w357] -> w352
                        stop <- w356 continue-if-true
                        n167 = call <userlib>:"GetStatus.vi"("error in (no error)"=w360) -> ("error out"=w357:errorcluster, "status"=w359:T19)  [unwired: 2 in, 1 out]
                        n168 = Equal?(x=w359, y=Error_Code_Enum_typedef."DRV_ACQUIRING") -> (x = y?=w356:bool)
                      }
                    }
                  }
                  n169 = local write "SaveStatus"(w336) -> ()
                }
                event "Exit": Value Change {
                  n170 = event-data() -> ()  [unwired: 1 in, 6 out]
                }
              }
            }
            frame "Exit" {
              n171 = local read "CoolerON"() -> (w372:T14)
              n172 = Unbundle By Name(w372) -> ("SetTemp"=w371:bool, "CoolerOn"=w370:bool)
              n173 = control-ref of="CurrentTemp"() -> (w369:refnum<vi>)
              n174 = control-ref of="ShutDown"() -> (w367:refnum<vi>)
              n175 = call "AndorShutdown.vi"("ShutDownRef"=w367, "CurrentTempRef"=w369, "error in"=w374, "CoolerON"=w370, "SetTemp"=w371) -> ("error out"=w373:errorcluster, "ShutDown"=w366:cluster{"CoolOff":bool, "ShutDown":bool}, "CurrentTemp"=w368:i32)  [unwired: 4 in]
              "ShutDown" <- w366
              n176 = local write "CurrentTemp"(w368) -> ()
              n177 = Unbundle By Name(w366) -> ("ShutDown"=w365:bool)  [unwired: 1 out]
            }
          }
        }
      }
    }
  }
